vi "Reversed By.vi"(11 "Relation in":refnum<class "Relation.lvclass">) -> (2 "Reversed By":string)   [LabVIEW 2022 SP3, in "Conditum.lvlib" / "Columns.lvlib" / "Relation.lvclass"]
uses:
  Relation.lvclass
  Relation.lvclass/Relation.ctl
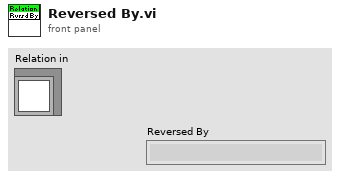
[diagram p1: front panel]
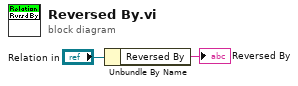
[diagram p0: block diagram]
diagram:
  n1 = Unbundle By Name("Relation in") -> ("Reversed By"=→"Reversed By":string)
